vi "Pause.vi"(8 "error in (no error)":errorcluster, 11 "Julabo FP-50 Settings In":T1) -> (0 "error out":errorcluster, 3 "Julabo FP-50 Settings Out":T1)   [LabVIEW 2021, in "HotCoil.lvlib"]
uses:
  HotCoil.lvlib
  HotCoil Settings.ctl
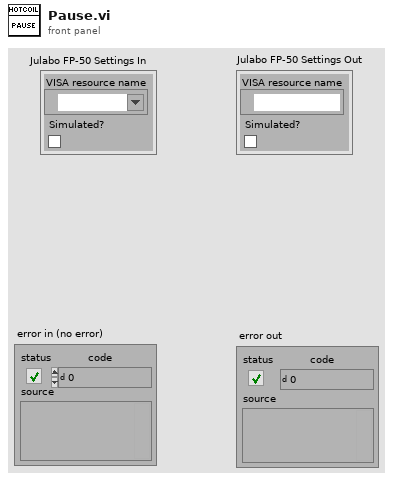
[diagram p1: front panel]
types:
  T1 = typedef "HotCoil.lvlib/HotCoil Settings.ctl" = cluster{"VISA resource name":refnum<visa-resource-name>, "Simulated?":bool}
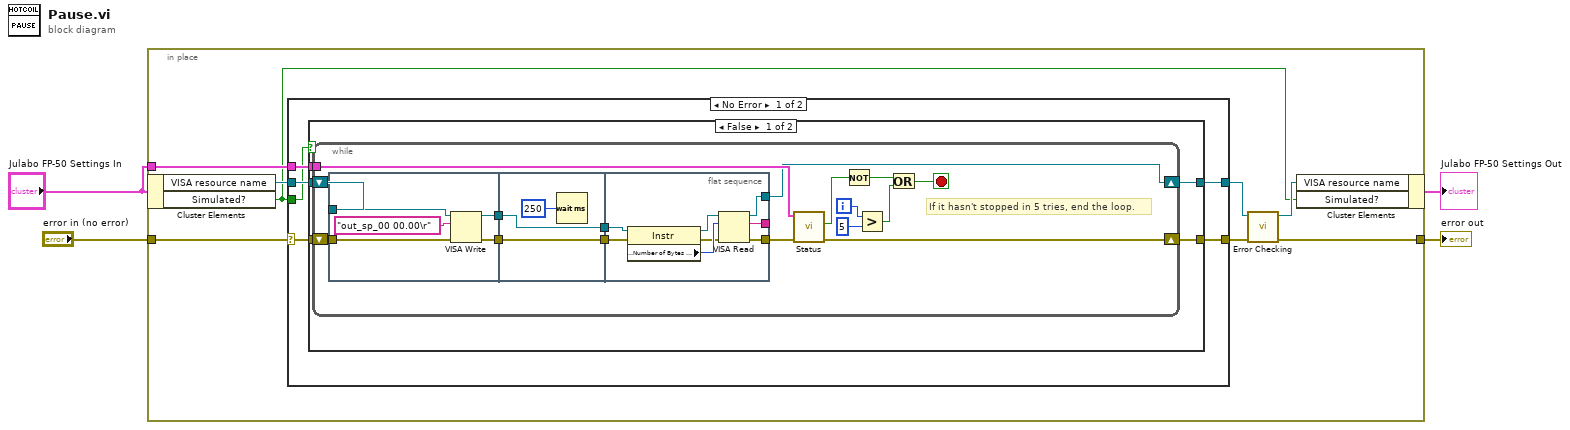
[diagram p0: block diagram]
diagram:
  n1 = in-place {
    in-place-border: "error in (no error)" -> [w12]
    in-place-border: [w9] -> w3
    in-place-border: "Julabo FP-50 Settings In" -> [w8]
    n2 = in-place-cluster #1("Julabo FP-50 Settings In") -> ("VISA resource name"=w7:refnum<visa-resource-name>, "Simulated?"=w5:bool)
    n3 = case shown="No Error" w12 {
      selector: w12 -> [w18 w59]
      tunnel: w8 -> [w15 _]
      tunnel: [w17 w59] -> w10
      tunnel: [w16 w58] -> w11
      tunnel: w7 -> [w14 w58]
      tunnel: w5 -> [w13 _]
      frame No Error {
        n4 = case shown="False" w13 {
          tunnel: w18 -> [w21 w57]
          tunnel: [w19 w57] -> w17
          tunnel: [w23 w56] -> w16
          tunnel: w14 -> [w22 w56]
          tunnel: w15 -> [w20 _]
          frame False {
            n5 = while {
              tunnel: w20 -> [w26]
              shift-right: [w24] -> w23
              shift-left: w22 -> [w28]
              shift-right: [w39] -> w19
              shift-left: w21 -> [w27]
              i -> [w37]
              stop <- w38 stop-if-true
              # "If it hasn't stopped in 5 tries, end the loop."
              n6 = flat-sequence {
                tunnel: w28 -> [w44]
                tunnel: [w43] -> w32
                tunnel: [w42] -> w31
                tunnel: w27 -> [w40]
                tunnel: w32 -> [w47]
                tunnel: [w47] -> w30
                tunnel: w31 -> [w46]
                tunnel: [w46] -> w29
                tunnel: [w55] -> w25
                tunnel: [w54] -> _
                tunnel: [w53] -> w24
                tunnel: w30 -> [w52]
                tunnel: w29 -> [w51]
                frame #0 {
                  n7 = VISA Write(VISA resource name=w44, write buffer="out_sp_00 00.00\r", error in (no error)=w40) -> (VISA resource name out=w43:refnum<visa-resource-name>, error out=w42:errorcluster)  [unwired: 1 out]
                }
                frame #1 {
                  n8 = Wait (ms)(milliseconds to wait=u32 250) -> ()  [unwired: 1 out]
                }
                frame #2 {
                  n9 = property class="Instr"(reference=w52, error in=w51) -> (reference out=w48:refnum<visa-resource-name>, error out=w49:errorcluster, "Serial Settings:Number of Bytes at Serial Port"=w50:u32)
                  n10 = VISA Read(VISA resource name=w48, byte count=w50, error in (no error)=w49) -> (VISA resource name out=w53:refnum<visa-resource-name>, read buffer=w54:string, error out=w55:errorcluster)  [unwired: 1 out]
                }
              }
              n11 = call "Status.vi"("error in (no error)"=w25, "HotCoil Settings In"=w26) -> ("error out"=w39:errorcluster, "Running"=w33:bool)  [unwired: 5 in, 3 out]
              n12 = Not(x=w33) -> (.not. x?=w34:bool)
              n13 = Greater?(x=w37, y=5) -> (0:w35:bool)
              n14 = Or(x=w34, y=w35) -> (x .or. y?=w38:bool)
            }
          }
          frame True {
          }
        }
      }
      frame Error {
      }
    }
    n15 = call "Error Checking.vi"("error in (no error)"=w10, "VISA resource name"=w11) -> ("error out"=w9:errorcluster, "VISA resource name"=w6:refnum<visa-resource-name>)  [unwired: 7 in, 1 out]
    n16 = in-place-cluster #1("VISA resource name"=w6, "Simulated?"=w5) -> (→"Julabo FP-50 Settings Out":T1)
  }
  "error out" <- w3
